vi "Init Sensor Queues.vi"() -> (3 "output cluster":T3)   [LabVIEW 2013]
doc: "This VI initalizes a series of queues which will be used to pass data between HB Sense and HB Think. The hindbrain pradigm is as follows: HB sense scrapes the simplest, most direct data possible, then puts that data in a queue as fast as it can. HB think pulls data from the queue, filters it if applicable, and writes the data to notifiers that MB and FB can see.\n\nIf new sensors are added, new queues should be created to pass the data to HB think.\n\nEric Schneider, April 2014"
uses:
  Data/TypeDefs/GPS-Compass Queue Cluster.ctl
  Data/TypeDefs/UTM Location.ctl
  Data/TypeDefs/WindData Queue Cluster.ctl
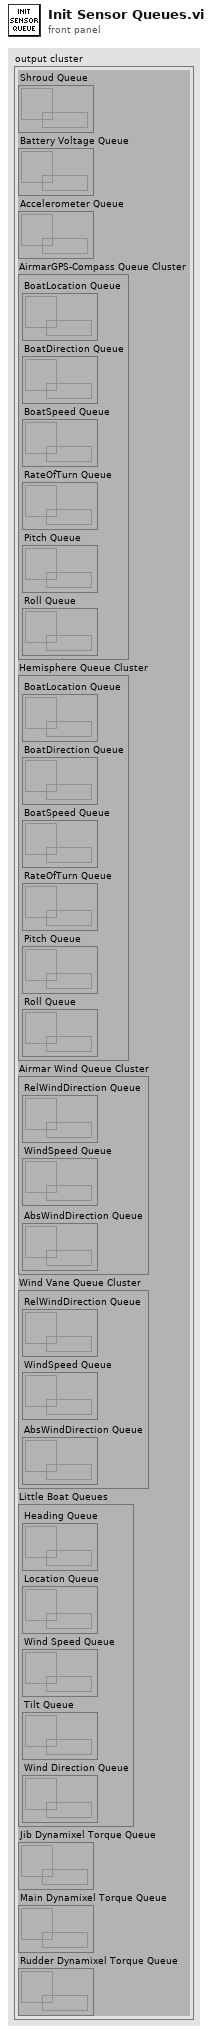
[diagram p1: front panel]
types:
  T1 = typedef "GPS-Compass Queue Cluster.ctl" = cluster{"BoatLocation Queue":refnum<queue>, "BoatDirection Queue":refnum<queue>, "BoatSpeed Queue":refnum<queue>, "RateOfTurn Queue":refnum<queue>, "Pitch Queue":refnum<queue>, "Roll Queue":refnum<queue>}
  T2 = typedef "WindData Queue Cluster.ctl" = cluster{"RelWindDirection Queue":refnum<queue>, "WindSpeed Queue":refnum<queue>, "AbsWindDirection Queue":refnum<queue>}
  T3 = cluster{"Shroud Queue":refnum<queue>, "Battery Voltage Queue":refnum<queue>, "Accelerometer Queue":refnum<queue>, "AirmarGPS-Compass Queue Cluster":T1, "Hemisphere Queue Cluster":T1, "Airmar Wind Queue Cluster":T2, "Wind Vane Queue Cluster":T2, "Little Boat Queues":cluster{"Heading Queue":refnum<queue>, "Location Queue":refnum<queue>, "Wind Speed Queue":refnum<queue>, "Tilt Queue":refnum<queue>, "Wind Direction Queue":refnum<queue>}, "Jib Dynamixel Torque Queue":refnum<queue>, "Main Dynamixel Torque Queue":refnum<queue>, "Rudder Dynamixel Torque Queue":refnum<queue>}
  T4 = cluster{"X-Axis Acceleration":dbl, "Y-Axis Acceleration":dbl, "Z-Axis Acceleration":dbl}
  T5 = cluster{"Heading Queue":refnum<queue>, "Location Queue":refnum<queue>, "Wind Speed Queue":refnum<queue>, "Tilt Queue":refnum<queue>, "Wind Direction Queue":refnum<queue>}
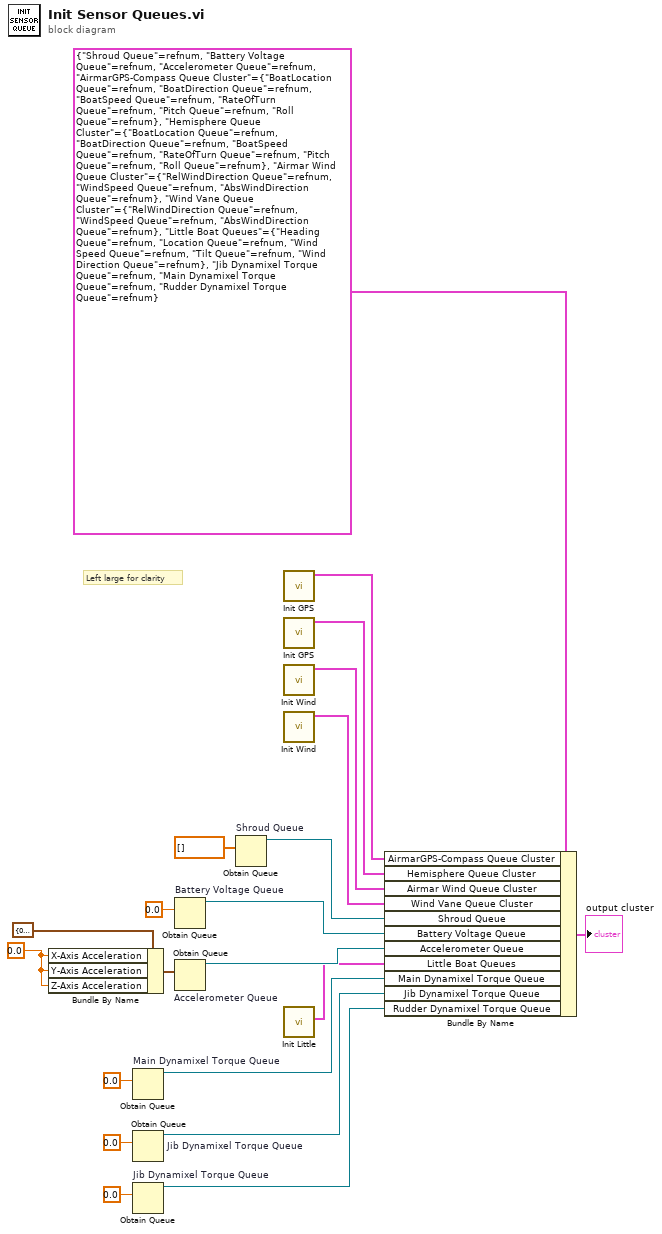
[diagram p0: block diagram]
diagram:
  w15 = 0.0 ("x+y")
  # "Left large for clarity"
  n1 = Bundle By Name(cluster=T4 {"X-Axis Acceleration"=0.0, "Y-Axis Acceleration"=0.0, "Z-Axis Acceleration"=0.0}, "X-Axis Acceleration"=w15, "Y-Axis Acceleration"=w15, "Z-Axis Acceleration"=w15) -> (w14:T4)
  n2 = Obtain Queue "Main Dynamixel Torque Queue"(element data type=0.0 ("x+y")) -> (queue out=w5:refnum<queue>)  [unwired: 4 in, 2 out]
  n3 = Obtain Queue "Jib Dynamixel Torque Queue"(element data type=0.0 ("x+y")) -> (queue out=w4:refnum<queue>)  [unwired: 4 in, 2 out]
  n4 = Obtain Queue "Jib Dynamixel Torque Queue"(element data type=0.0 ("x+y")) -> (queue out=w2:refnum<queue>)  [unwired: 4 in, 2 out]
  n5 = Obtain Queue "Battery Voltage Queue"(element data type=0.0 ("x+y")) -> (queue out=w18:refnum<queue>)  [unwired: 4 in, 2 out]
  n6 = Obtain Queue "Accelerometer Queue"(element data type=w14) -> (queue out=w13:refnum<queue>)  [unwired: 4 in, 2 out]
  n7 = Obtain Queue "Shroud Queue"(element data type=dbl[] []) -> (queue out=w20:refnum<queue>)  [unwired: 4 in, 2 out]
  n8 = call "Init GPS.vi"() -> ("GPS-Compass Queue Cluster"=w12:T1)  [unwired: 11 in]
  n9 = call "Init GPS.vi"() -> ("GPS-Compass Queue Cluster"=w11:T1)  [unwired: 11 in]
  n10 = call "Init Wind.vi"() -> ("Wind Queue Cluster"=w10:T2)  [unwired: 11 in]
  n11 = call "Init Wind.vi"() -> ("Wind Queue Cluster"=w9:T2)  [unwired: 11 in]
  n12 = call "Init Little.vi"() -> ("Little Boat Queues"=w8:T5)  [unwired: 11 in]
  n13 = Bundle By Name(cluster=T3 {"Shroud Queue"=refnum, "Battery Voltage Queue"=refnum, "Accelerometer Queue"=refnum, "AirmarGPS-Compass Queue Cluster"={"BoatLocation Queue"=refnum, "BoatDirection Queue"=refnum, "BoatSpeed Queue"=refnum, "RateOfTurn Queue"=refnum, "Pitch Queue"=refnum, "Roll Queue"=refnum}, "Hemisphere Queue Cluster"={"BoatLocation Queue"=refnum, "BoatDirection Queue"=refnum, "BoatSpeed Queue"=refnum, "RateOfTurn Queue"=refnum, "Pitch Queue"=refnum, "Roll Queue"=refnum}, "Airmar Wind Queue Cluster"={"RelWindDirection Queue"=refnum, "WindSpeed Queue"=refnum, "AbsWindDirection Queue"=refnum}, "Wind Vane Queue Cluster"={"RelWindDirection Queue"=refnum, "WindSpeed Queue"=refnum, "AbsWindDirection Queue"=refnum}, "Little Boat Queues"={"Heading Queue"=refnum, "Location Queue"=refnum, "Wind Speed Queue"=refnum, "Tilt Queue"=refnum, "Wind Direction Queue"=refnum}, "Jib Dynamixel Torque Queue"=refnum, "Main Dynamixel Torque Queue"=refnum, "Rudder Dynamixel Torque Queue"=refnum} ("output cluster"), "AirmarGPS-Compass Queue Cluster"=w12, "Hemisphere Queue Cluster"=w11, "Airmar Wind Queue Cluster"=w10, "Wind Vane Queue Cluster"=w9, "Shroud Queue"=w20, "Battery Voltage Queue"=w18, "Accelerometer Queue"=w13, "Little Boat Queues"=w8, "Main Dynamixel Torque Queue"=w5, "Jib Dynamixel Torque Queue"=w4, "Rudder Dynamixel Torque Queue"=w2) -> (→"output cluster":T3)
